vi "SuperVI3_0.vi"() -> ()   [LabVIEW 2021]
uses:
  <vilib>/MakerHub/LINX/Public/Peripherals/Digital/Digital Write 1 Chan.vi
  <vilib>/MakerHub/LINX/Public/Peripherals/Digital/Digital Write N Chans.vi
  <vilib>/MakerHub/LINX/Private/Local IO/LinxDigitalWrite.vi
  <vilib>/MakerHub/LINX/Public/Utilities/Check Channel.vi
  <vilib>/MakerHub/LINX/Public/Utilities/Open Serial.vi
  <vilib>/MakerHub/LINX/Private/Utilties/Generate Error.vi
  <vilib>/MakerHub/LINX/LMH-LINX.lvlib
panel:
  in  "?":bool
  in  "Vary Threshold":dbl=7.0
  out "Average Noise":dbl
  in  "?":bool
  out "Calibration":dbl[](graph)
  in  "Start Wavelength":dbl=364.05
  in  "Wavelength/Step":dbl=0.45
  out "Transmission (%)":cluster{dbl[], "appended array":dbl[]}(graph)
  out "Absorption (%)":cluster{dbl[], "appended array":dbl[]}(graph)
  out "FILTER":cluster{dbl[], "appended array":dbl[]}(graph)
  out "LED":cluster{dbl[], "appended array":dbl[]}(graph)
  in  "End Green":dbl=550.0
  in  "End Blue":dbl=260.0
  in  "?":bool
  in  "Number of Filters":i32
  in  "Calibrate":bool
  in  "STOP":bool
  in  "?":bool
  in  "?":bool
  in  "?":bool
  in  "M1":bool
  in  "M0":bool
  in  "Motor steps":i32
  out "error out":errorcluster
  in  "Serial Port":refnum<visa-resource-name>="N/A"
  in  "error in (no error)":errorcluster
  # "Function & M0 & M1\n ----------------------\nFull  Step:       0         0\n1/2   Step:       1         0\n1/8   Step:       0         1\n1/16 Step:       1         1"
  # "------------------------------------------------------------\n                                           HOW TO\n                                         CALIBRATE\n------------------------------------------------------------\n1. Block the LED to measure the average noise intensity\n2. Select the amount of Filters you wanna use to calibrate\n3. Start the program with\nthe 'Calibrate' button pressed (Let it measure)\n4. Take out what was blocking the light, put in the first filter and\npress the 'START CALIBRATION button (Let it  measure)\n5. Put the rest of the filters and let it measure. Press\nthe 'NEXT FILTER' button after each measurement \n6. Once all filters have been measured, take out the\n filters and press the 'END CALIBRATION' button\n7. Now you can measure the samples with the measured\ncalibration"
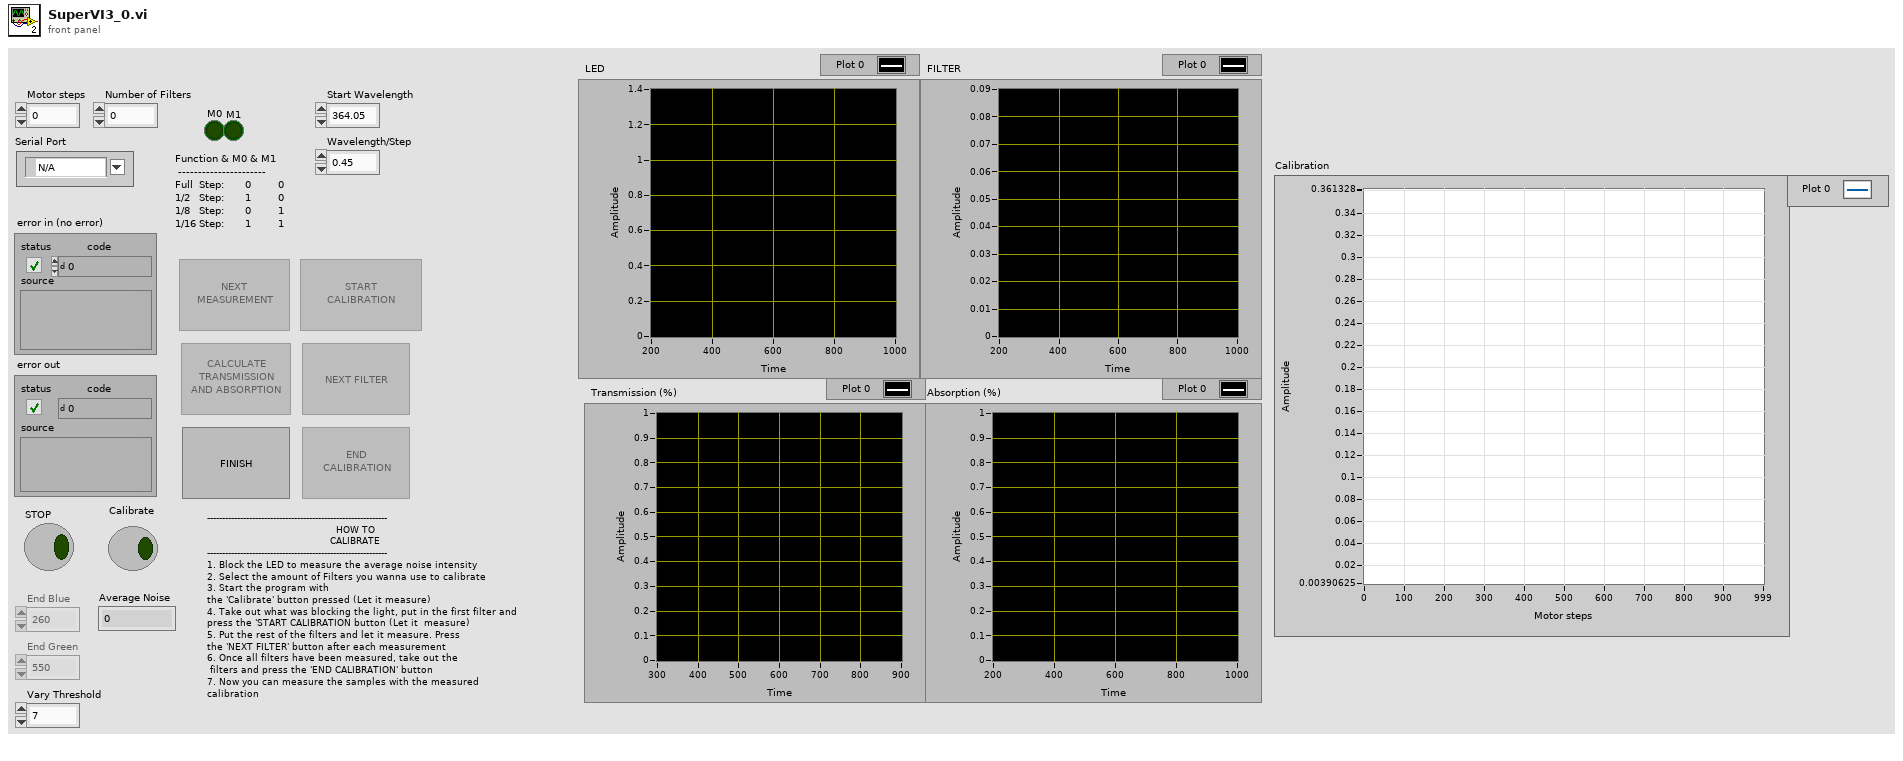
[diagram p1: front panel]
types:
  T1 = typedef "LMH-LINX.lvlib/LINX Ref.ctl" = cluster{"IO":T2, "Interface":T3, "LINX Device Config":T4}
  T2 = typedef "LMH-LINX.lvlib/Platform.ctl" = enum16{"Remote", "Local"}
  T3 = typedef "LMH-LINX.lvlib/Interface.ctl" = enum16{"Serial", "TCP"}
  T4 = typedef "LMH-LINX.lvlib/Device.lvlib/LINX Device Config.ctl" = cluster{"Interface":T3, "COM Port":refnum<visa-resource-name>, "TCP Configuration":T5, "Device Family":u8, "Device ID":u8, "Device Name":string, "TCP Ref":refnum<k5>, "Channels":T6}
  T5 = typedef "LMH-LINX.lvlib/Device.lvlib/TCP Config.ctl" = cluster{"IP Address":string, "Port":u16}
  T6 = typedef "LMH-LINX.lvlib/Channels.ctl" = cluster{"DI":u8[], "DO":u8[], "AI":u8[], "AO":u8[], "PWM":u8[], "QE":u8[], "UART":u8[], "I2C 2":u8[], "SPI":u8[], "CAN":u8[], "Servo":u8[], "AI Ref (V)":dbl, "AI Resolution (Bits)":u8, "AO Ref (V)":dbl, "AO Resolution (Bits)":u8}
  T7 = enum8{"Enabled", "Disabled", "Disabled and Grayed Out"}
  T8 = cluster{"appended array":dbl[], "appended array":dbl[]}
  T9 = cluster{"appended array":dbl[], "appended array 2":dbl[]}
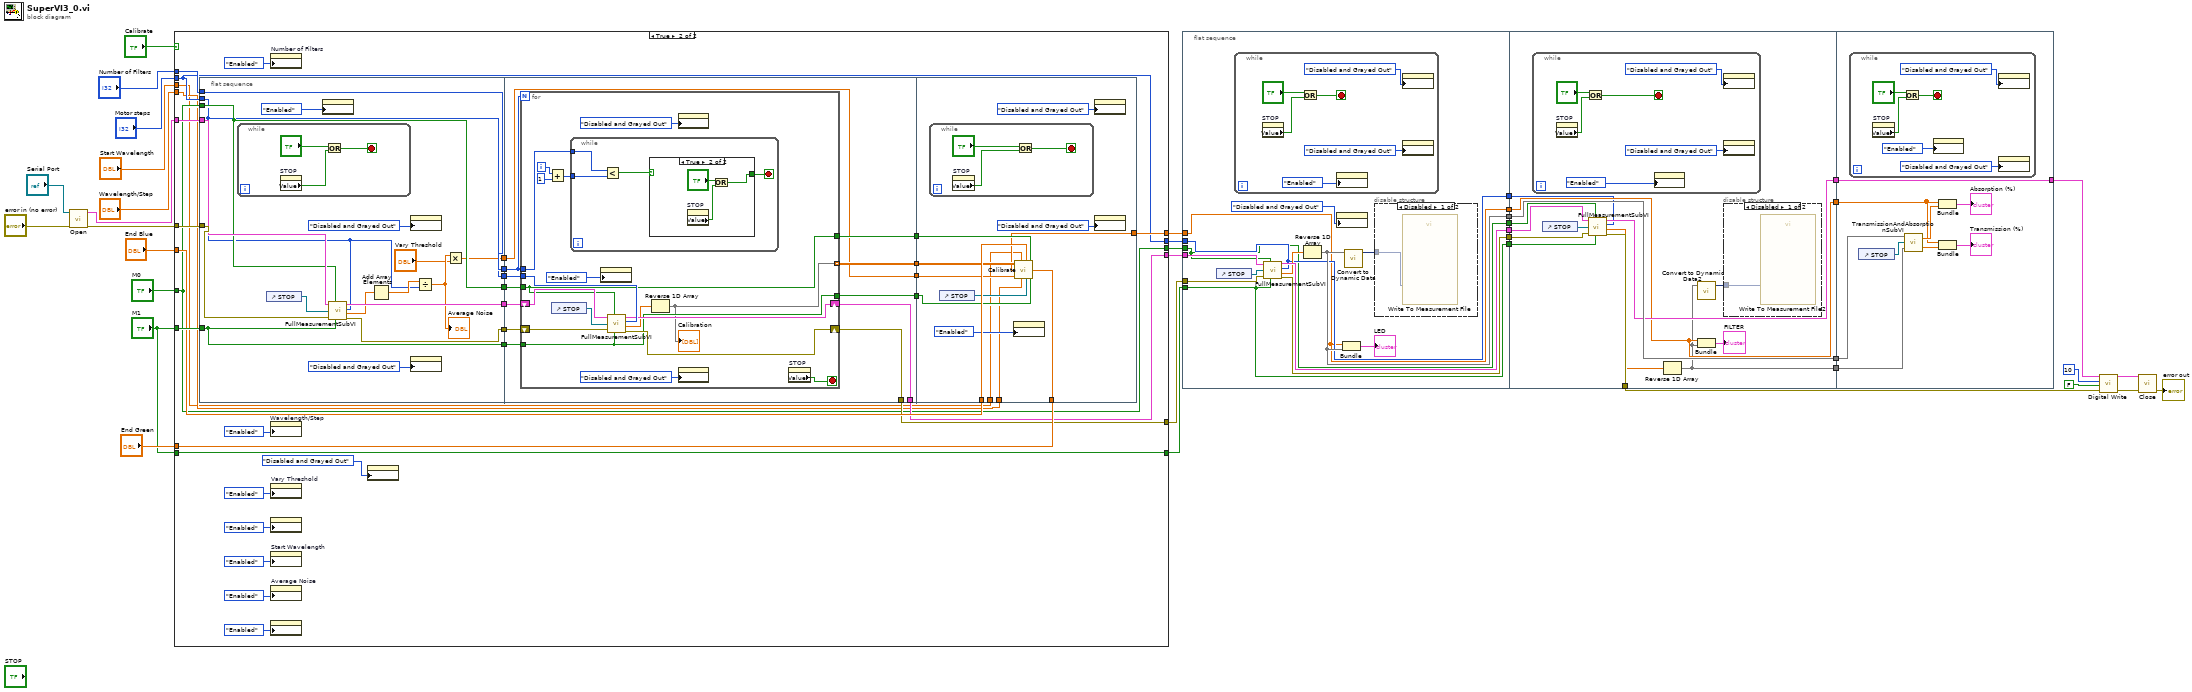
[diagram p0: block diagram]
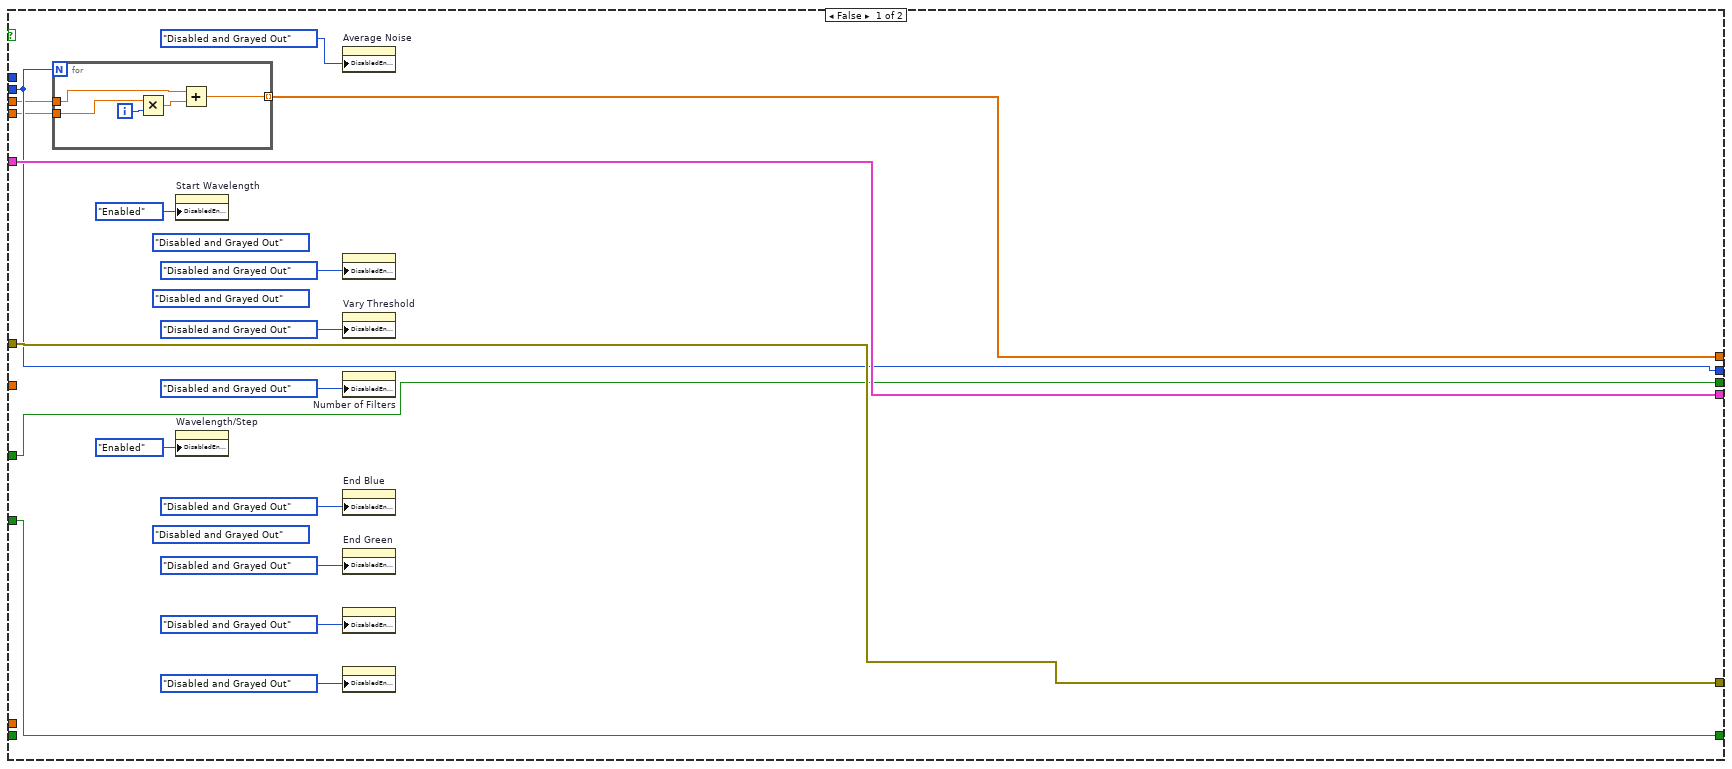
[diagram p2: hidden frame]
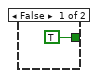
[diagram p3: hidden frame]
diagram:
  n1 = call-poly <vilib>:"Open.vi"("Error In"="error in (no error)", "Serial Port"="Serial Port") -> ("Error Out"=w19:errorcluster, "LINX Resource"=w21:T1)  [unwired: 7 in, 1 out]
  n2 = case shown="True" "Calibrate" {
    tunnel: w21 -> [w55 w92]
    tunnel: [w55 w85] -> w20
    tunnel: w19 -> [w54 w91]
    tunnel: [w54 w86] -> w18
    tunnel: "Motor steps" -> [w49 w77]
    tunnel: [w49 w77] -> w16
    tunnel: [w53 w75] -> w15
    tunnel: "M0" -> [w53 w75]
    tunnel: "M1" -> [w52 w90]
    tunnel: [w52 w76] -> w13
    tunnel: "Number of Filters" -> [_ w93]
    tunnel: [w39 w82] -> w9
    tunnel: "End Blue" -> [_ w88]
    tunnel: "End Green" -> [_ w87]
    tunnel: "Wavelength/Step" -> [w48 w63]
    tunnel: "Start Wavelength" -> [w40 w61]
    tunnel: "M1" -> [_ w76]
    frame False {
      (unwired) T7."Disabled and Grayed Out" ("Disabled")
      (unwired) T7."Disabled and Grayed Out" ("Disabled")
      (unwired) T7."Disabled and Grayed Out" ("Disabled")
      n3 = for {
        N: w49 -> [_]
        tunnel: w48 -> [w59]
        tunnel: w40 -> [w57]
        tunnel: [w56] -> w39 mode=indexing
        i -> [w60]
        n4 = Multiply(x=w59, y=w60) -> (x*y=w58:dbl)
        n5 = Add(x=w57, y=w58) -> (x+y=w56:dbl)
      }
      n6 = property on="Start Wavelength" class="DigNum (strict)"("DisabledEnum"=T7."Enabled" ("Disabled")) -> ()  [unwired: 2 in, 2 out]
      n7 = property on="Wavelength/Step" class="DigNum (strict)"("DisabledEnum"=T7."Enabled" ("Disabled")) -> ()  [unwired: 2 in, 2 out]
      n8 = property on="Average Noise" class="DigNum (strict)"("DisabledEnum"=T7."Disabled and Grayed Out" ("Disabled")) -> ()  [unwired: 2 in, 2 out]
      n9 = property class="Bool"("DisabledEnum"=T7."Disabled and Grayed Out" ("Disabled")) -> ()  [unwired: 2 in, 2 out]
      n10 = property on="Vary Threshold" class="DigNum (strict)"("DisabledEnum"=T7."Disabled and Grayed Out" ("Disabled")) -> ()  [unwired: 2 in, 2 out]
      n11 = property on="Number of Filters" class="DigNum (strict)"("DisabledEnum"=T7."Disabled and Grayed Out" ("Disabled")) -> ()  [unwired: 2 in, 2 out]
      n12 = property on="End Blue" class="DigNum (strict)"("DisabledEnum"=T7."Disabled and Grayed Out" ("Disabled")) -> ()  [unwired: 2 in, 2 out]
      n13 = property on="End Green" class="DigNum (strict)"("DisabledEnum"=T7."Disabled and Grayed Out" ("Disabled")) -> ()  [unwired: 2 in, 2 out]
      n14 = property class="Bool"("DisabledEnum"=T7."Disabled and Grayed Out" ("Disabled")) -> ()  [unwired: 2 in, 2 out]
      n15 = property class="Bool"("DisabledEnum"=T7."Disabled and Grayed Out" ("Disabled")) -> ()  [unwired: 2 in, 2 out]
    }
    frame True {
      n16 = flat-sequence {
        tunnel: w77 -> [w100]
        tunnel: w90 -> [w103]
        tunnel: w75 -> [w104]
        tunnel: w91 -> [w110]
        tunnel: w92 -> [w108]
        tunnel: w93 -> [w106]
        tunnel: [w106] -> w74
        tunnel: [w107] -> w73
        tunnel: [w109] -> w72
        tunnel: [w104] -> w71
        tunnel: [w103] -> w70
        tunnel: [w100] -> w69
        tunnel: [w99] -> w67
        tunnel: [w120] -> w89
        tunnel: [w119] -> w86
        tunnel: [w118] -> w85
        tunnel: [w117] -> w84
        tunnel: [w116] -> w83
        tunnel: w74 -> [w114]
        tunnel: w73 -> [w125]
        tunnel: w72 -> [w124]
        tunnel: w71 -> [w123]
        tunnel: w70 -> [w122]
        tunnel: w69 -> [w121]
        tunnel: [w115] -> w68
        tunnel: w67 -> [w115]
        tunnel: w89 -> [w159]
        tunnel: w88 -> [w164]
        tunnel: w87 -> [w163]
        tunnel: w84 -> [w161]
        tunnel: w83 -> [w160]
        tunnel: [w158] -> w82
        tunnel: w68 -> [w157]
        tunnel: w63 -> [w153]
        tunnel: w61 -> [w152]
        frame #0 {
          n17 = while {
            stop <- w112 stop-if-true
            n18 = property on="STOP" class="Bool (strict)"() -> ("Value"=w111:bool)  [unwired: 2 in, 2 out]
            n19 = Or(x="?", y=w111) -> (x .or. y?=w112:bool)
          }
          n20 = control-ref of="STOP"() -> (w105:refnum<vi>)
          n21 = property class="Bool"("DisabledEnum"=T7."Enabled" ("Disabled")) -> ()  [unwired: 2 in, 2 out]
          n22 = call "FullMeasurementSubVI.vi"("LINX Resource"=w108, "M0"=w104, "Stop REF"=w105, "error in (no error)"=w110, "M1"=w103, "Motor steps"=w100) -> ("LINX Resource 2"=w107:T1, "Array"=w102:dbl[], "error out"=w109:errorcluster)
          n23 = Add Array Elements(numeric array=w102) -> (sum=w101:dbl)
          n24 = property class="Bool"("DisabledEnum"=T7."Disabled and Grayed Out" ("Disabled")) -> ()  [unwired: 2 in, 2 out]
          n25 = property class="Bool"("DisabledEnum"=T7."Disabled and Grayed Out" ("Disabled")) -> ()  [unwired: 2 in, 2 out]
          n26 = Divide(x=w101, y=w100) -> (x/y=w98:dbl)
          "Average Noise" <- w98
          n27 = Multiply(x=w98, y="Vary Threshold") -> (x*y=w99:dbl)
        }
        frame #1 {
          n28 = for {
            N: w114 -> [_]
            tunnel: w123 -> [w136]
            tunnel: w122 -> [w135]
            tunnel: w121 -> [w139]
            tunnel: [w130] -> w120 mode=indexing
            shift-right: [w137] -> w118
            shift-left: w125 -> [w142]
            shift-right: [w138] -> w119
            shift-left: w124 -> [w140]
            tunnel: [w136] -> w117
            tunnel: [w135] -> w116
            tunnel: w114 -> [w129]
            i -> [w128]
            stop <- w143 stop-if-true
            n29 = Add(x=w128, y=1) -> (x+y=w127:i32)
            n30 = control-ref of="STOP"() -> (w141:refnum<vi>)
            n31 = while {
              tunnel: w129 -> [w145]
              tunnel: w127 -> [w144]
              stop <- w147 stop-if-true
              n32 = Less?(x=w145, y=w144) -> (x < y?=w146:bool)
              n33 = case shown="True" w146 {
                tunnel: [TRUE w151] -> w147
                frame False {
                }
                frame True {
                  n34 = property on="STOP" class="Bool (strict)"() -> ("Value"=w149:bool)  [unwired: 2 in, 2 out]
                  n35 = Or(x="?", y=w149) -> (x .or. y?=w151:bool)
                }
              }
            }
            n36 = property class="Bool"("DisabledEnum"=T7."Enabled" ("Disabled")) -> ()  [unwired: 2 in, 2 out]
            n37 = call "FullMeasurementSubVI.vi"("LINX Resource"=w142, "M0"=w136, "Stop REF"=w141, "error in (no error)"=w140, "M1"=w135, "Motor steps"=w139) -> ("LINX Resource 2"=w137:T1, "Array"=w131:dbl[], "error out"=w138:errorcluster)
            n38 = Reverse 1D Array(array=w131) -> (reversed array=w130:dbl[])
            "Calibration" <- w130
            n39 = property class="Bool"("DisabledEnum"=T7."Disabled and Grayed Out" ("Disabled")) -> ()  [unwired: 2 in, 2 out]
            n40 = property class="Bool"("DisabledEnum"=T7."Disabled and Grayed Out" ("Disabled")) -> ()  [unwired: 2 in, 2 out]
            n41 = property on="STOP" class="Bool (strict)"() -> ("Value"=w143:bool)  [unwired: 2 in, 2 out]
          }
        }
        frame #2 {
          n42 = while {
            stop <- w166 stop-if-true
            n43 = property on="STOP" class="Bool (strict)"() -> ("Value"=w165:bool)  [unwired: 2 in, 2 out]
            n44 = Or(x="?", y=w165) -> (x .or. y?=w166:bool)
          }
          n45 = control-ref of="STOP"() -> (w162:refnum<vi>)
          n46 = property class="Bool"("DisabledEnum"=T7."Enabled" ("Disabled")) -> ()  [unwired: 2 in, 2 out]
          n47 = call "Calibrate.vi"("Array 2"=w159, "Starting Wavelength"=w152, "Threshold"=w157, "Wavelength/Step"=w153, "End Blue"=w164, "M0"=w161, "End Green"=w163, "STOP REF"=w162, "M1"=w160) -> ("appended array"=w158:dbl[])
          n48 = property class="Bool"("DisabledEnum"=T7."Disabled and Grayed Out" ("Disabled")) -> ()  [unwired: 2 in, 2 out]
          n49 = property class="Bool"("DisabledEnum"=T7."Disabled and Grayed Out" ("Disabled")) -> ()  [unwired: 2 in, 2 out]
        }
      }
      n50 = property on="Number of Filters" class="DigNum (strict)"("DisabledEnum"=T7."Enabled" ("Disabled")) -> ()  [unwired: 2 in, 2 out]
      n51 = property on="Wavelength/Step" class="DigNum (strict)"("DisabledEnum"=T7."Enabled" ("Disabled")) -> ()  [unwired: 2 in, 2 out]
      n52 = property on="Vary Threshold" class="DigNum (strict)"("DisabledEnum"=T7."Enabled" ("Disabled")) -> ()  [unwired: 2 in, 2 out]
      n53 = property class="Bool"("DisabledEnum"=T7."Enabled" ("Disabled")) -> ()  [unwired: 2 in, 2 out]
      n54 = property on="Start Wavelength" class="DigNum (strict)"("DisabledEnum"=T7."Enabled" ("Disabled")) -> ()  [unwired: 2 in, 2 out]
      n55 = property on="Average Noise" class="DigNum (strict)"("DisabledEnum"=T7."Enabled" ("Disabled")) -> ()  [unwired: 2 in, 2 out]
      n56 = property class="Bool"("DisabledEnum"=T7."Enabled" ("Disabled")) -> ()  [unwired: 2 in, 2 out]
      n57 = property class="Bool"("DisabledEnum"=T7."Disabled and Grayed Out" ("Disabled")) -> ()  [unwired: 2 in, 2 out]
    }
  }
  n58 = flat-sequence {
    tunnel: [w173] -> w29
    tunnel: [w180] -> w27
    tunnel: [w178] -> w26
    tunnel: w20 -> [w176]
    tunnel: w18 -> [w175]
    tunnel: w16 -> [w172]
    tunnel: w15 -> [w170]
    tunnel: w13 -> [w171]
    tunnel: w9 -> [w169]
    tunnel: [w169] -> w8
    tunnel: [w172] -> w3
    tunnel: [w171] -> w2
    tunnel: [w170] -> w1
    tunnel: [w202] -> w30
    tunnel: w29 -> [w202]
    tunnel: [w192] -> w28
    tunnel: w27 -> [w200]
    tunnel: w26 -> [w199]
    tunnel: [w198] -> w25
    tunnel: [w197] -> w23
    tunnel: w8 -> [w193]
    tunnel: [w193] -> w7
    tunnel: w3 -> [w191]
    tunnel: w2 -> [w190]
    tunnel: w1 -> [w189]
    tunnel: w30 -> [w217]
    tunnel: w28 -> [w216]
    tunnel: [w215] -> w24
    tunnel: w23 -> [w215]
    tunnel: w7 -> [w210]
    frame #0 {
      n59 = control-ref of="STOP"() -> (w177:refnum<vi>)
      n60 = while {
        stop <- w185 stop-if-true
        n61 = property on="STOP" class="Bool (strict)"() -> ("Value"=w183:bool)  [unwired: 2 in, 2 out]
        n62 = Or(x="?", y=w183) -> (x .or. y?=w185:bool)
        n63 = property class="Bool"("DisabledEnum"=T7."Enabled" ("Disabled")) -> ()  [unwired: 2 in, 2 out]
        n64 = property class="Bool"("DisabledEnum"=T7."Disabled and Grayed Out" ("Disabled")) -> ()  [unwired: 2 in, 2 out]
        n65 = property class="Bool"("DisabledEnum"=T7."Disabled and Grayed Out" ("Disabled")) -> ()  [unwired: 2 in, 2 out]
      }
      n66 = call "FullMeasurementSubVI.vi"("LINX Resource"=w176, "M0"=w170, "Stop REF"=w177, "error in (no error)"=w175, "M1"=w171, "Motor steps"=w172) -> ("LINX Resource 2"=w180:T1, "Array"=w179:dbl[], "error out"=w178:errorcluster)
      n67 = Reverse 1D Array(array=w179) -> (reversed array=w173:dbl[])
      n68 = property class="Bool"("DisabledEnum"=T7."Disabled and Grayed Out" ("Disabled")) -> ()  [unwired: 2 in, 2 out]
      n69 = Bundle("appended array"=w169, w173) -> (→"LED":cluster{"appended array":dbl[], dbl[]})  [unwired: 1 in]
      n70 = call "Convert to Dynamic Data"("Array"=w173) -> ("Dynamic Data Type"=w181:dynamicdata)  [unwired: 3 in]
      n71 = disable-structure shown="Disabled" {
        disable-tunnel: w181 -> [w182 _]
        frame Disabled {
          n72 = call "Write To Measurement File"("Signals"=w182) -> ()  [unwired: 16 in, 3 out]
        }
        frame Enabled {
        }
      }
    }
    frame #1 {
      n73 = while {
        stop <- w205 stop-if-true
        n74 = property on="STOP" class="Bool (strict)"() -> ("Value"=w206:bool)  [unwired: 2 in, 2 out]
        n75 = Or(x="?", y=w206) -> (x .or. y?=w205:bool)
        n76 = property class="Bool"("DisabledEnum"=T7."Enabled" ("Disabled")) -> ()  [unwired: 2 in, 2 out]
        n77 = property class="Bool"("DisabledEnum"=T7."Disabled and Grayed Out" ("Disabled")) -> ()  [unwired: 2 in, 2 out]
        n78 = property class="Bool"("DisabledEnum"=T7."Disabled and Grayed Out" ("Disabled")) -> ()  [unwired: 2 in, 2 out]
      }
      n79 = control-ref of="STOP"() -> (w195:refnum<vi>)
      n80 = call "FullMeasurementSubVI.vi"("LINX Resource"=w200, "M0"=w189, "Stop REF"=w195, "error in (no error)"=w199, "M1"=w190, "Motor steps"=w191) -> ("LINX Resource 2"=w197:T1, "Array"=w196:dbl[], "error out"=w198:errorcluster)
      n81 = Reverse 1D Array(array=w196) -> (reversed array=w192:dbl[])
      n82 = Bundle("appended array"=w193, w192) -> (→"FILTER":cluster{"appended array":dbl[], dbl[]})  [unwired: 1 in]
      n83 = call "Convert to Dynamic Data2"("Array"=w192) -> ("Dynamic Data Type"=w201:dynamicdata)  [unwired: 3 in]
      n84 = disable-structure shown="Disabled" {
        disable-tunnel: w201 -> [w203 _]
        frame Disabled {
          n85 = call "Write To Measurement File2"("Signals"=w203) -> ()  [unwired: 16 in, 3 out]
        }
        frame Enabled {
        }
      }
    }
    frame #2 {
      n86 = while {
        stop <- w220 stop-if-true
        n87 = property on="STOP" class="Bool (strict)"() -> ("Value"=w219:bool)  [unwired: 2 in, 2 out]
        n88 = Or(x="?", y=w219) -> (x .or. y?=w220:bool)
        n89 = property class="Bool"("DisabledEnum"=T7."Enabled" ("Disabled")) -> ()  [unwired: 2 in, 2 out]
        n90 = property class="Bool"("DisabledEnum"=T7."Disabled and Grayed Out" ("Disabled")) -> ()  [unwired: 2 in, 2 out]
        n91 = property class="Bool"("DisabledEnum"=T7."Disabled and Grayed Out" ("Disabled")) -> ()  [unwired: 2 in, 2 out]
      }
      n92 = control-ref of="STOP"() -> (w218:refnum<vi>)
      n93 = call "TransmissionAndAbsorptionSubVI.vi"("array 2"=w216, "Stop REF"=w218, "array"=w217) -> ("appended array 2"=w211:dbl[], "appended array"=w212:dbl[])
      n94 = Bundle("appended array"=w210, "appended array"=w212) -> (→"Absorption (%)":T8)  [unwired: 1 in]
      n95 = Bundle("appended array"=w210, "appended array 2"=w211) -> (→"Transmission (%)":T9)  [unwired: 1 in]
    }
  }
  n96 = call-poly <vilib>:"Digital Write.vi"("Error In"=w25, "Output Value"=FALSE, "DO Channel"=u8 10, "LINX Resource"=w24) -> ("Error Out"=w31:errorcluster, "LINX Resource"=w32:T1)  [unwired: 6 in]
  n97 = call <vilib>:"Close.vi"("Error In"=w31, "LINX Resource"=w32) -> ("Error Out"=→"error out":errorcluster)  [unwired: 9 in]
